vi "Save data to HDF5.vi"(4 "Photodiode channel":i32=1, 6 "PMT Channel":i32, 7 "coefficient info":T1(array[cluster]) {"offset" format="%^_6e"; "gain" format="%^_6e"; "reserved 1" format="%^_6e"; "reserved 2" format="%^_6e"}, 8 "error in (no error)":errorcluster, 9 "Save data?":bool, 11 "HDF5 Dataset Ref":T2) -> (0 "error out":errorcluster, 3 "HDF5 Dataset out":T2)   [LabVIEW 2018]
uses:
  <vilib>/UPVI/lvhdf5/library.llb/HDF5 Ref.ctl
  <vilib>/UPVI/lvhdf5/dataset.llb/Append Element(s) to Dataset (Variant).vi
  <vilib>/UPVI/lvhdf5/dataset.llb/Append Element(s) to Dataset.xnode
panel:
  in  "wfm":i16[][](array[numeric])
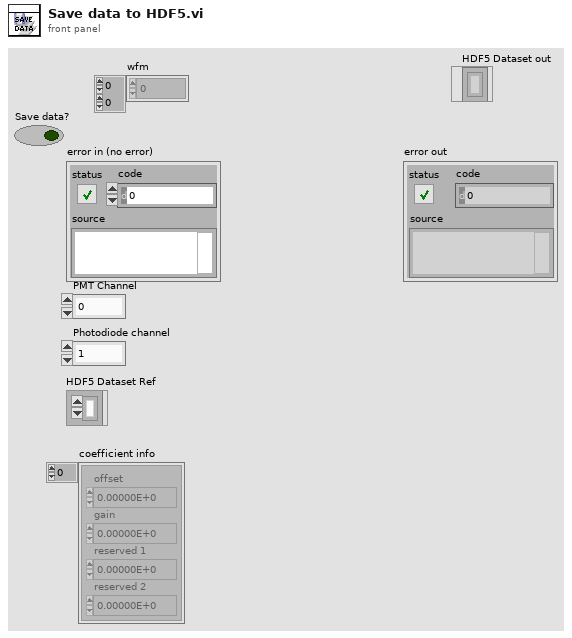
[diagram p1: front panel]
types:
  T1 = cluster{"offset":dbl, "gain":dbl, "reserved 1":dbl, "reserved 2":dbl}[]
  T2 = typedef "HDF5 Ref.ctl" = refnum<k1>
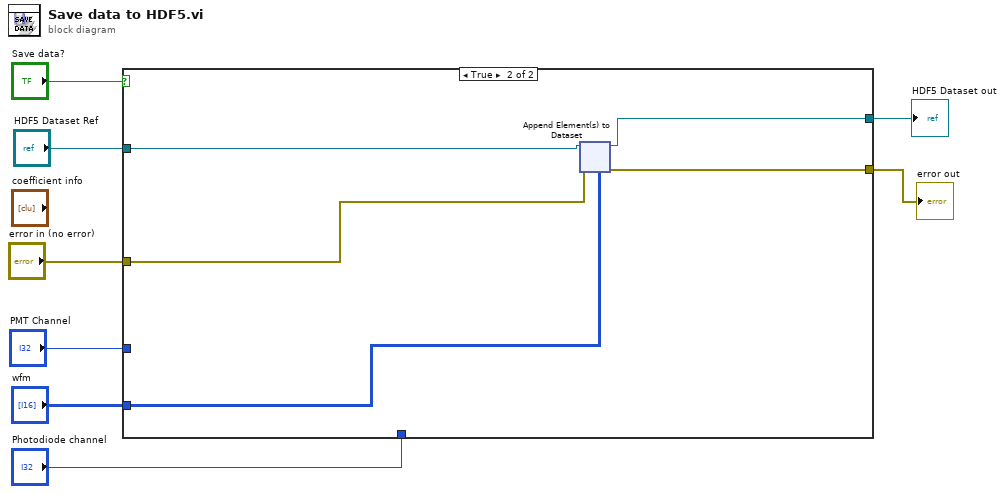
[diagram p0: block diagram]
diagram:
  n1 = case shown="True" "Save data?" {
    tunnel: "wfm" -> [_ w11]
    tunnel: "error in (no error)" -> [w10 w13]
    tunnel: [w10 w14] -> w6
    tunnel: "HDF5 Dataset Ref" -> [w9 w15]
    tunnel: "PMT Channel" -> [_ _]
    tunnel: "Photodiode channel" -> [_ _]
    tunnel: [w9 w12] -> w2
    frame False {
    }
    frame True {
      n2 = xnode "Append Element(s) to Dataset"("HDF5 Dataset Ref"=w15, "error in (no error)"=w13, "Data Element(s)"=w11) -> ("HDF5 Dataset out"=w12:T2, "error out"=w14:errorcluster)  [unwired: 1 in, 2 out]
    }
  }
  "error out" <- w6
  "HDF5 Dataset out" <- w2
